vi "svl_Peak Level with IC.vi"(8 "error in (no error)":errorcluster, 9 "processing state":T1(ring), 10 "initial soundLevel":dbl format="%.2f", 11 "scaled signal":waveform(dbl)={"t0"=timestamp(0 s since 1904-01-01), "dt"=0.0, "Y"=[]}) -> (0 "error out":errorcluster, 2 "final soundLevel":dbl format="%.2f")   [LabVIEW 2017]
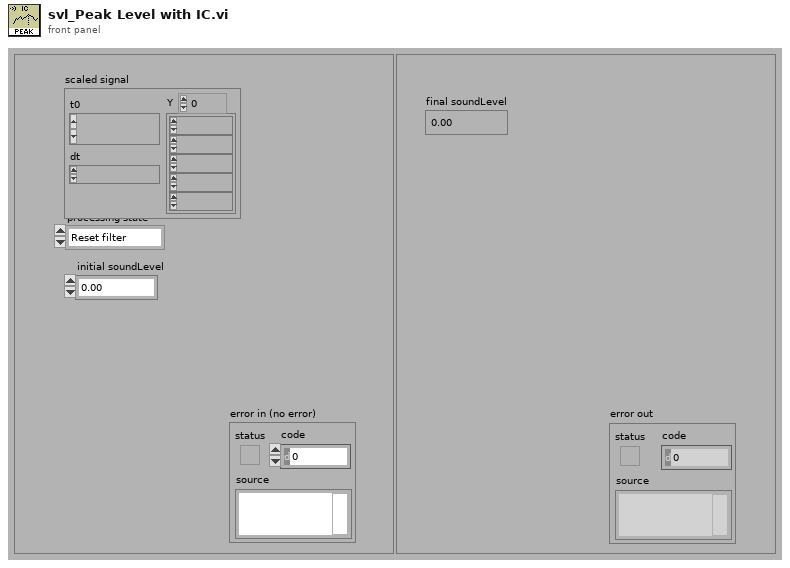
[diagram p1: front panel]
types:
  T1 = enum16{"Reset filter", "Restart averaging", "Continue processing"}
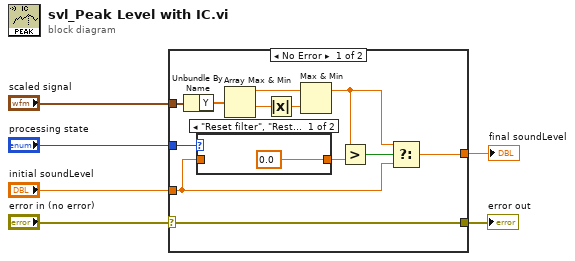
[diagram p0: block diagram]
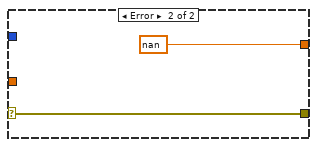
[diagram p3: hidden frame]
diagram:
  n1 = case shown="No Error" "error in (no error)" {
    selector: "error in (no error)" -> [w18 w22]
    tunnel: [w18 w22] -> w4
    tunnel: "scaled signal" -> [w8 _]
    tunnel: "processing state" -> [w17 _]
    tunnel: "initial soundLevel" -> [w11 _]
    tunnel: [w12 nan ("soundLevel")] -> w6
    frame No Error {
      n2 = Unbundle By Name(w8) -> ("Y"=w7:dbl[])
      n3 = case shown="\"Reset filter\", \"Restart averaging\", Default" w17 {
        tunnel: w11 -> [_ w20]
        tunnel: [0.0 ("t") w20] -> w10
        frame "Reset filter", "Restart averaging", Default {
        }
        frame "Continue processing" {
        }
      }
      n4 = Array Max & Min(array=w7) -> (max value=w15:dbl, min value=w16:dbl)  [unwired: 2 out]
      n5 = Absolute Value(x=w16) -> (abs(x)=w14:dbl)
      n6 = Max & Min(x=w15, y=w14) -> (max(x,y)=w9:dbl)  [unwired: 1 out]
      n7 = Greater?(x=w9, y=w10) -> (0:w13:bool)
      n8 = Select(t=w9, s=w13, f=w11) -> (s? t:f=w12:dbl)
    }
    frame Error {
    }
  }
  "final soundLevel" <- w6
  "error out" <- w4
